vi "SWERVE_DRIVE_ACQUIRE.vi"(6 "Pass_Through_Time":dbl=-1.0 format="%33.4f", 8 "error in (no error)":errorcluster, 10 "GyroDevRef":T1={"DevStatus"={"status"=FALSE, "code"=0, "source"=""}, "Analog Channel"=enum."AI 1", "Gain (VoltsPerDegree/Second)"=0.0, "Gyro Type"=enum."Analog", "Handle"=0, "SPI Bus"=enum."Invalid", "Device Found"=FALSE, "Sample Rate"=1.0, "Calibrate On Open"=FALSE, "Offset"=0.0} {"Sample Rate" min=0.25 max=100.0 step=0.25}, 11 "Swerve IO Reference":T4[](array[typedef])) -> (0 "error out":errorcluster)   [LabVIEW 2019]
uses:
  SWERVE_DRIVE_MODULE_TYPDEF.ctl
  <vilib>/Rock Robotics/WPI/MotorControl/WPI_MotorControlDeviceRef.ctl
  <vilib>/Rock Robotics/WPI/MotorControl/WPI_MotorControlType.ctl
  <vilib>/Rock Robotics/SystemInterfaces/DIO/FPGA_DIOPWMChannel.ctl
  <vilib>/Rock Robotics/WPI/PWM/WPI_PWMDeadband.ctl
  <vilib>/Rock Robotics/SystemInterfaces/DIO/FPGA_DIOChannel.ctl
  <vilib>/Rock Robotics/WPI/Encoder/WPI_EncoderDevRef.ctl
  <vilib>/Rock Robotics/SystemInterfaces/Encoder/FPGA_EncoderIdx.ctl
  <vilib>/Rock Robotics/SystemInterfaces/Counter/FPGA_CounterCtrSystemIndex.ctl
  <vilib>/Rock Robotics/WPI/Encoder/WPI_EncoderType.ctl
  <vilib>/Rock Robotics/WPI/Gyro/WPI_GyroDevRef.ctl
  <vilib>/Rock Robotics/SystemInterfaces/AI/FPGA_AIChannel.ctl
  <vilib>/Rock Robotics/SystemInterfaces/spilib/spi_bus.ctl
  <vilib>/Rock Robotics/WPI/ThirdParty/JAS_Junk/TrajLib/VI/Util_GetTime_U32.vi
  <vilib>/Rock Robotics/WPI/ThirdParty/JAS_Junk/TrajLib/MathUtil_InputModulus.vi
  SWERVE_DRIVE_GLOBALS.vi
  <vilib>/Rock Robotics/WPI/ThirdParty/JAS_Junk/TrajLib/VI/Util_GetTime_U64.vi
  <vilib>/Rock Robotics/WPI/ThirdParty/JAS_Junk/TrajLib/Trajectory_Library.lvlib
panel:
  # "Analog"
  # "XRS"
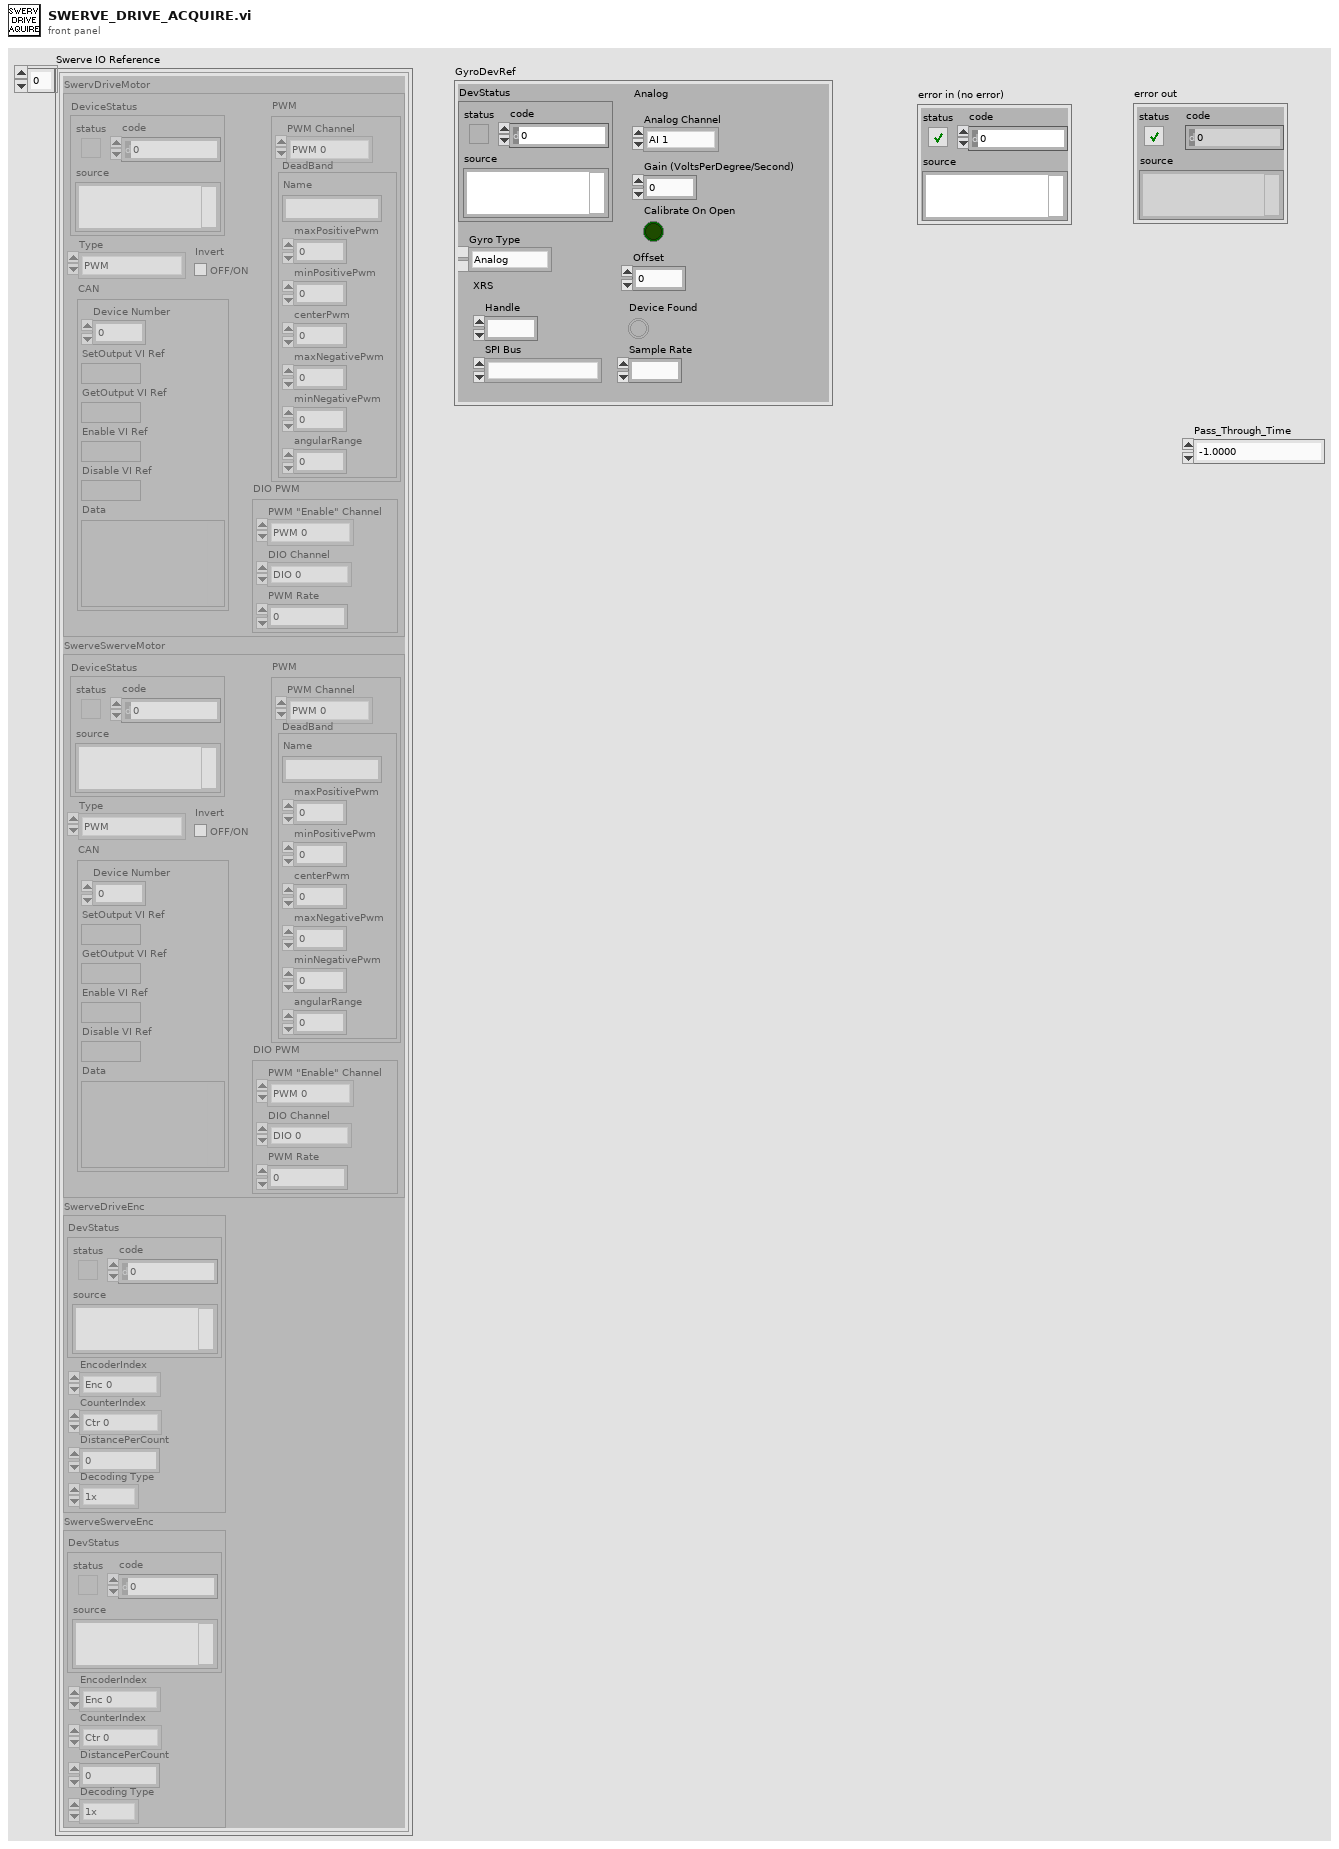
[diagram p1: front panel]
types:
  T1 = typedef "WPI_GyroDevRef.ctl" = cluster{"DevStatus":errorcluster, "Analog Channel":T2, "Gain (VoltsPerDegree/Second)":dbl, "Gyro Type":enum16{"Analog", "XRS450"}, "Handle":i32, "SPI Bus":T3, "Device Found":bool, "Sample Rate":dbl, "Calibrate On Open":bool, "Offset":dbl}
  T2 = typedef "FPGA_AIChannel.ctl" = enum8{"AI 0", "AI 1", "AI 2", "AI 3", "AI MXP 0", "AI MXP 1", "AI MXP 2", "AI MXP 3", "Invalid"}
  T3 = typedef "spi_bus.ctl" = enum16{"SPI On-Board, CS0", "SPI On-Board, CS1", "SPI On-Board, CS2", "SPI On-Board, CS3", "SPI MXP", "Invalid"}
  T4 = typedef "SWERVE_DRIVE_MODULE_TYPDEF.ctl" = cluster{"SwervDriveMotor":T5, "SwerveSwerveMotor":T5, "SwerveDriveEnc":T10, "SwerveSwerveEnc":T10}
  T5 = typedef "WPI_MotorControlDeviceRef.ctl" = cluster{"DeviceStatus":errorcluster, "Type":T6, "PWM":cluster{"PWM Channel":T7, "DeadBand":T8}, "CAN":cluster{"Device Number":u8, "SetOutput VI Ref":variant, "GetOutput VI Ref":variant, "Enable VI Ref":variant, "Disable VI Ref":variant, "Data":variant}, "Invert":bool, "DIO PWM":cluster{"PWM \"Enable\" Channel":T7, "DIOChannel":T9, "PWM Rate":dbl}}
  T6 = typedef "WPI_MotorControlType.ctl" = enum16{"PWM", "CAN", "DIO PWM"}
  T7 = typedef "FPGA_DIOPWMChannel.ctl" = enum8{"PWM 0", "PWM 1", "PWM 2", "PWM 3", "PWM 4", "PWM 5", "PWM 6", "PWM 7", "PWM 8", "PWM 9", "PWM MXP 0", "PWM MXP 1", "PWM MXP 2", "PWM MXP 3", "PWM MXP 4", "PWM MXP 5", "PWM MXP 6", "PWM MXP 7", "PWM MXP 8", "PWM MXP 9", "Invalid"}
  T8 = typedef "WPI_PWMDeadband.ctl" = cluster{"Name":string, "maxPositivePwm":i32, "minPositivePwm":i32, "centerPwm":i32, "maxNegativePwm":i32, "minNegativePwm":i32, "angularRange":u16}
  T9 = typedef "FPGA_DIOChannel.ctl" = enum8{"DIO 0", "DIO 1", "DIO 2", "DIO 3", "DIO 4", "DIO 5", "DIO 6", "DIO 7", "DIO 8", "DIO 9", "DIO MXP 0", "DIO MXP 1", "DIO MXP 2", "DIO MXP 3", "DIO MXP 4", "DIO MXP 5", "DIO MXP 6", "DIO MXP 7", "DIO MXP 8", "DIO MXP 9", "DIO MXP 10", "DIO MXP 11", "DIO MXP 12", "DIO MXP 13", "DIO MXP 14", "DIO MXP 15", "SPI Port CS1", "SPI Port CS2", "SPI Port CS3", "SPI Port MISO", "SPI Port MOSI", "Invalid"}
  T10 = typedef "WPI_EncoderDevRef.ctl" = cluster{"DevStatus":errorcluster, "EncoderIndex":T11, "CounterIndex":T12, "DistancePerCount":dbl, "Decoding Type":T13}
  T11 = typedef "FPGA_EncoderIdx.ctl" = enum8{"Enc 0", "Enc 1", "Enc 2", "Enc 3", "Enc 4", "Enc 5", "Enc 6", "Enc 7", "Invalid"}
  T12 = typedef "FPGA_CounterCtrSystemIndex.ctl" = enum8{"Ctr 0", "Ctr 1", "Ctr 2", "Ctr 3", "Ctr 4", "Ctr 5", "Ctr 6", "Ctr 7", "Invalid"}
  T13 = typedef "WPI_EncoderType.ctl" = enum16{"1x", "2x", "4x"}
  T14 = typedef "Trajectory_Library.lvlib/SWERVE_DRIVE_KINEMATICS.ctl" = cluster{"NumModules":i32, "InverseKinematics":T15, "ForwardKinematics":T15, "Modules":T16[], "PrevCoR":T16, "SavedModuleStates":T17[]}
  T15 = typedef "NI_Matrix.lvlib/RealMatrix.ctl" = dbl[][]
  T16 = typedef "Trajectory_Library.lvlib/TRANSLATION2D.ctl" = cluster{"X":dbl, "Y":dbl}
  T17 = typedef "Trajectory_Library.lvlib/SWERVE_DRIVE_MODULE_STATE.ctl" = cluster{"Speed":dbl, "Angle":T18}
  T18 = typedef "Trajectory_Library.lvlib/ROTATION2D.ctl" = cluster{"VALUE":dbl, "COS":dbl, "SIN":dbl}
  T19 = typedef "Trajectory_Library.lvlib/SWERVE_DRIVE_MODULE_POSITION.ctl" = cluster{"Distance":dbl, "Angle":T18, "P":bool}
  T20 = typedef "Trajectory_Library.lvlib/CHASSIS_SPEEDS.ctl" = cluster{"vX":dbl, "vY":dbl, "vOmega":dbl}
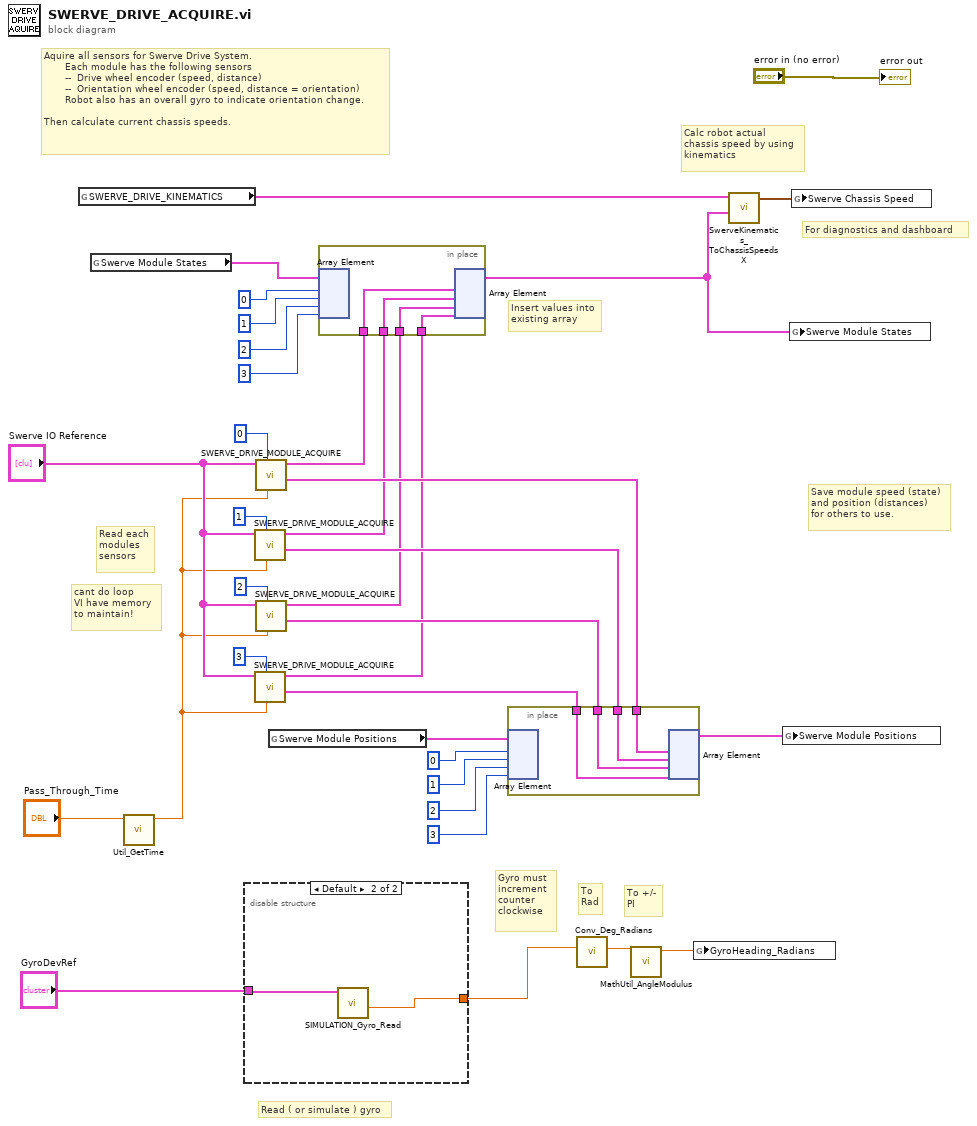
[diagram p0: block diagram]
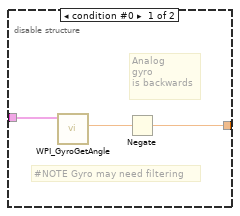
[diagram p2: hidden frame]
diagram:
  # "Insert values into\nexisting array"
  # "For diagnostics and dashboard"
  # "Read each\nmodules\nsensors"
  # "Gyro must\nincrement \ncounter\nclockwise"
  # "To +/-\nPI"
  # "To\nRad"
  # "Read ( or simulate ) gyro"
  # "Aquire all sensors for Swerve Drive System.\n       Each module has the following sensors\n       --  Drive wheel encoder (speed, distance)\n       --  Orientation wheel encoder (speed, distance = orientation)\n       Robot also has an overall gyro to indicate orientation change.\n\nThen calculate current chassis speeds."
  # "Calc robot actual\nchassis speed by using\nkinematics"
  # "Save module speed (state)\nand position (distances)\nfor others to use."
  # "cant do loop\nVI have memory\nto maintain!"
  n1 = global read "SWERVE_DRIVE_GLOBALS.vi" "SWERVE_DRIVE_KINEMATICS"() -> (w30:T14)
  n2 = global read "SWERVE_DRIVE_GLOBALS.vi" "Swerve Module States"() -> (w8:T17[])
  n3 = call <vilib>:"Util_GetTime.vi"("Pass_Through_Time"="Pass_Through_Time") -> ("FPGA_Time_Seconds"=w23:dbl)  [unwired: 8 in, 2 out]
  n4 = disable-structure shown="Default" {
    disable-tunnel: "GyroDevRef" -> [w37 w39]
    disable-tunnel: [w35 w38] -> w1
    frame condition #0 {
      # "Analog\ngyro\nis backwards"
      # "#NOTE Gyro may need filtering"
      n5 = call <vilib>:"WPI_GyroGetAngle.vi"("GyroDevRef"=w37) -> ("Angle"=w36:dbl)  [unwired: 6 in, 4 out]
      n6 = Negate(x=w36) -> (-x=w35:dbl)
    }
    frame condition #1 (active) {
      n7 = call "SIMULATION_Gyro_Read.vi"("GyroDevRef"=w39) -> ("Gyro_Cont_Deg"=w38:dbl)  [unwired: 10 in]
    }
  }
  n8 = call "SWERVE_DRIVE_MODULE_ACQUIRE.vi"("Pass_Through_Time"=w23, "Swerve Module Inx"=1, "Swerve Module TypDef"="Swerve IO Reference") -> ("SWERVE DRIVE MODULE POSITION"=w16:T19, "Swerve Module State"=w6:T17)  [unwired: 7 in]
  n9 = call "SWERVE_DRIVE_MODULE_ACQUIRE.vi"("Pass_Through_Time"=w23, "Swerve Module Inx"=3, "Swerve Module TypDef"="Swerve IO Reference") -> ("SWERVE DRIVE MODULE POSITION"=w14:T19, "Swerve Module State"=w4:T17)  [unwired: 7 in]
  n10 = call "SWERVE_DRIVE_MODULE_ACQUIRE.vi"("Pass_Through_Time"=w23, "Swerve Module Inx"=0, "Swerve Module TypDef"="Swerve IO Reference") -> ("SWERVE DRIVE MODULE POSITION"=w17:T19, "Swerve Module State"=w7:T17)  [unwired: 7 in]
  n11 = call "SWERVE_DRIVE_MODULE_ACQUIRE.vi"("Pass_Through_Time"=w23, "Swerve Module Inx"=2, "Swerve Module TypDef"="Swerve IO Reference") -> ("SWERVE DRIVE MODULE POSITION"=w15:T19, "Swerve Module State"=w5:T17)  [unwired: 7 in]
  n12 = global read "SWERVE_DRIVE_GLOBALS.vi" "Swerve Module Positions"() -> (w18:T19[])
  n13 = in-place {
    in-place-border: w7 -> [w43]
    in-place-border: w6 -> [w42]
    in-place-border: w5 -> [w41]
    in-place-border: w4 -> [w40]
    n14 = in-place-array #1(w8, 0, 1, 2, 3) -> ()  [unwired: 4 out]
    n15 = in-place-array #1(w43, w42, w41, w40) -> (w3:T17[])  [unwired: 4 out]
  }
  n16 = in-place {
    in-place-border: w17 -> [w47]
    in-place-border: w16 -> [w46]
    in-place-border: w15 -> [w45]
    in-place-border: w14 -> [w44]
    n17 = in-place-array #2(w18, 0, 1, 2, 3) -> ()  [unwired: 4 out]
    n18 = in-place-array #2(w47, w46, w45, w44) -> (w13:T19[])  [unwired: 4 out]
  }
  n19 = call <vilib>:"Conv_Deg_Radians.vi"("Degress"=w1) -> ("Radians"=w33:dbl)  [unwired: 10 in]
  n20 = call <vilib>:"MathUtil_AngleModulus.vi"("InputAngle"=w33) -> ("ModulsAngle"=w32:dbl)  [unwired: 10 in]
  n21 = global write "SWERVE_DRIVE_GLOBALS.vi" "GyroHeading_Radians"(w32) -> ()
  n22 = call <vilib>:"SwerveKinematics_ToChassisSpeedsX.vi"("WheelStates"=w3, "in SWERVE_DRIVE_KINEMATICS"=w30) -> ("Chassis Speed"=w31:T20)  [unwired: 9 in]
  n23 = global write "SWERVE_DRIVE_GLOBALS.vi" "Swerve Module Positions"(w13) -> ()
  n24 = global write "SWERVE_DRIVE_GLOBALS.vi" "Swerve Module States"(w3) -> ()
  n25 = global write "SWERVE_DRIVE_GLOBALS.vi" "Swerve Chassis Speed"(w31) -> ()
  "error out" <- "error in (no error)"
